vi "DualEncodersReadoutCore(NI-DAQmx).vi"(8 "error in":errorcluster, 9 "Position Out Queue":refnum<queue>, 10 "ctrl queue in":refnum<queue>) -> (0 "error out":errorcluster)   [LabVIEW 2014, in "EncoderReadout(NI-DAQmx).lvlib"]
uses:
  EncoderReadout(NI-DAQmx).lvlib
  VI/Encoder_State.ctl
  VI/EncoderReadout_Configs.ctl
  VI/EncoderReadout_PrivateStats.ctl
  <vilib>/Utility/error.llb/DialogType.ctl
  <vilib>/DAQmx/configure/timing.llb/DAQmx Timing (Sample Clock).vi
  <vilib>/DAQmx/read.llb/DAQmx Read (Counter 1D DBL 1Chan NSamp).vi
  <vilib>/Utility/error.llb/Error Cluster From Error Code.vi
  <vilib>/ErrorRing/Error Ring.xnode
  <resource>/objmgr/daqmx.rc
  <userlib>/Utility/ErrorLog_lib.lvlib
panel:
  out "ChangeDetect.Overflowed":bool
  out "start cts":i32
  out "TotalSampPerChanAcquired":dbl format="%#.2f"
  out "CurrReadPos":dbl
  out "AvailSampPerChan":u32
  out "PreGetPosition":dbl format="%_19f"
  out "flushbufffer":dbl format="%_19f"
  out "flush buffer":dbl[](graph)
  out "data":dbl[](graph)
  out "post flush buffer":i32
  out "pre-flush buffer":u32
  in  "SetPositionButton":bool
  out "elements":T1[](array[typedef])
  in  "Continuous":bool
  out "acqu. time":dbl
  out "pos get position":dbl format="%_19f"
  out "trans. start stamp":dbl format="%_19f"
  out "ctr_getpos":i32
  in  "SetPosition":dbl[](array[numeric])=[0.0, 0.0]
  in  "Get Configs":bool
  in  "StartAll":bool
  out "Core#":i32
  out "LiveStat":T2
  in  "EncoderReadout_Config":T3={"Mode"=enum."NSamples", "# Channels"=1, "# Samples"=128, "SyncSource"="/cDAQ1Mod3/PFI3", "Timeout (s)"=3600.0}
  out "Graph":dbl[][](graph)
  in  "Reset":bool
  in  "Close":bool
  in  "Open":bool
  in  "Quit":bool
  in  "GetPositions":bool
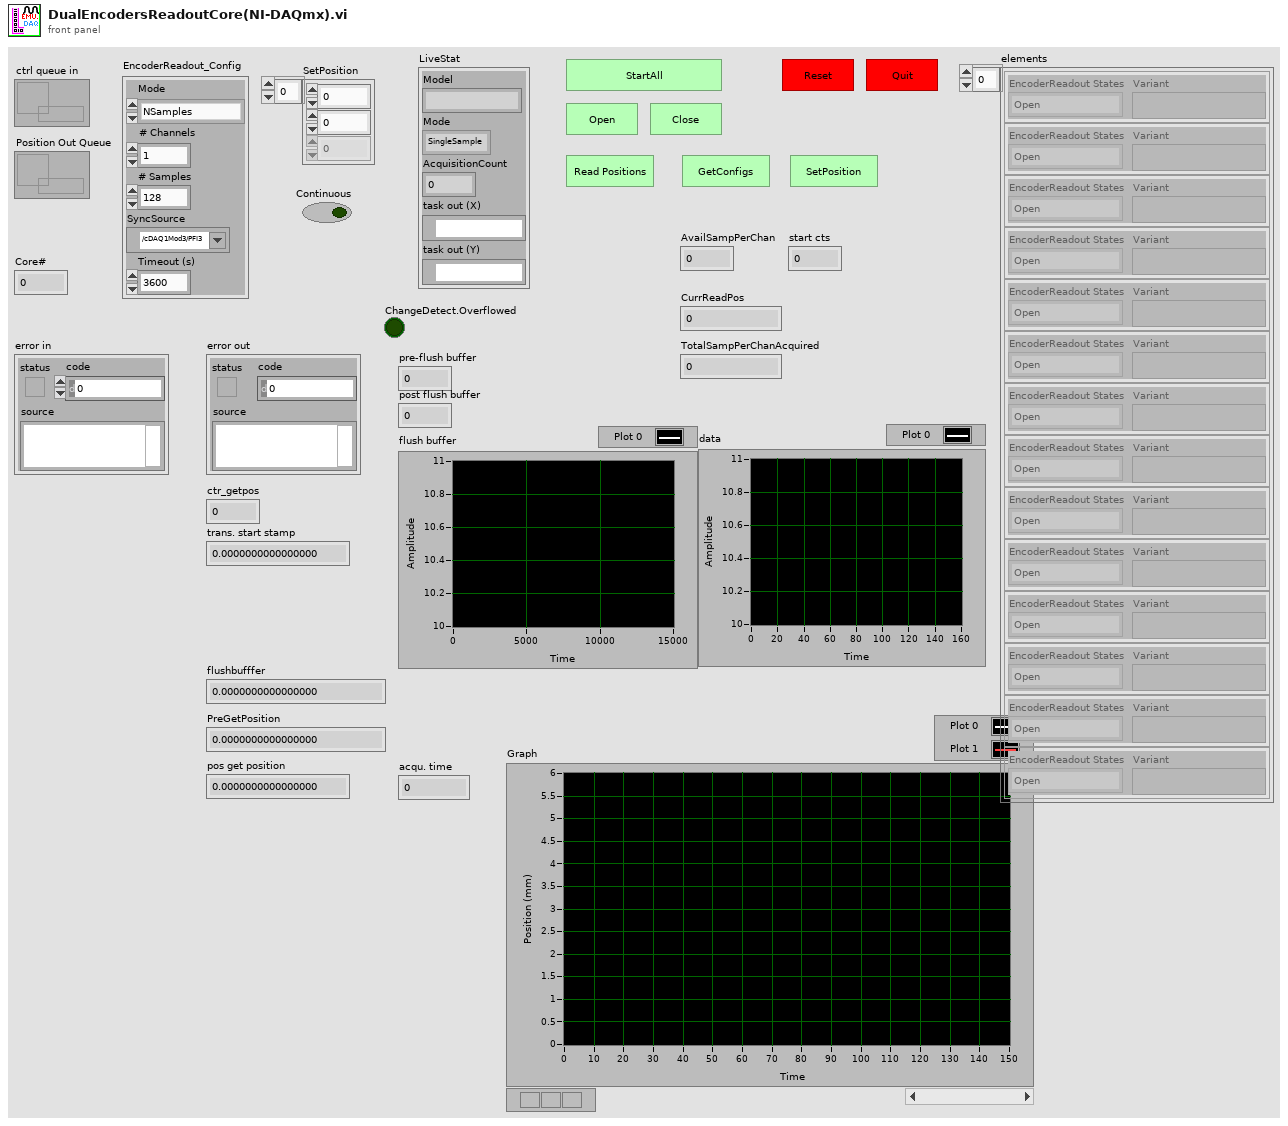
[diagram p1: front panel]
types:
  T1 = typedef "EncoderReadout(NI-DAQmx).lvlib/Encoder_State.ctl" = cluster{"EncoderReadout States":enum16{"Open", "Close", "Quit", "SetPosition", "SetPointsNum", "SetSyncChannel", "Start(Flush)", "GetPositions", "QueryStatus", "SetTimeout", "SetMode", "SetSignalOutputBuffer", "GetConfigs", "Wait", "Clear", "Stop", "FlushBuffer"}, "Variant":variant}
  T2 = typedef "EncoderReadout(NI-DAQmx).lvlib/EncoderReadout_PrivateStats.ctl" = cluster{"Model":string, "Mode":enum16{"SingleSample", "NSamples", "Continuous"}, "AcquisitionCount":i32, "task out (X)":refnum<k21>, "task out (Y)":refnum<k21>}
  T3 = typedef "EncoderReadout(NI-DAQmx).lvlib/EncoderReadout_Configs.ctl" = cluster{"Mode":enum16{"SingleSample", "NSamples", "Continuous"}, "# Channels":i32, "# Samples":i32, "SyncSource":tag, "Timeout (s)":dbl}
  T4 = typedef "DialogType.ctl" = u16
  T5 = cluster{"tickcount":u32, "Position":dbl[][], "Flag":enum16{"Normal", "MultiRecStart", "MultiRecEnd", "Reserved1", "Reserved2", "Reserved3"}}
  T6 = enum16{"Open", "Close", "Quit", "SetPosition", "SetPointsNum", "SetSyncChannel", "Start(Flush)", "GetPositions", "QueryStatus", "SetTimeout", "SetMode", "SetSignalOutputBuffer", "GetConfigs", "Wait", "Clear", "Stop", "FlushBuffer"}
  T7 = typedef "EncoderReadout_Configs.ctl" = cluster{"Mode":enum16{"SingleSample", "NSamples", "Continuous"}, "# Channels":i32, "# Samples":i32, "SyncSource":tag, "Timeout (s)":dbl}
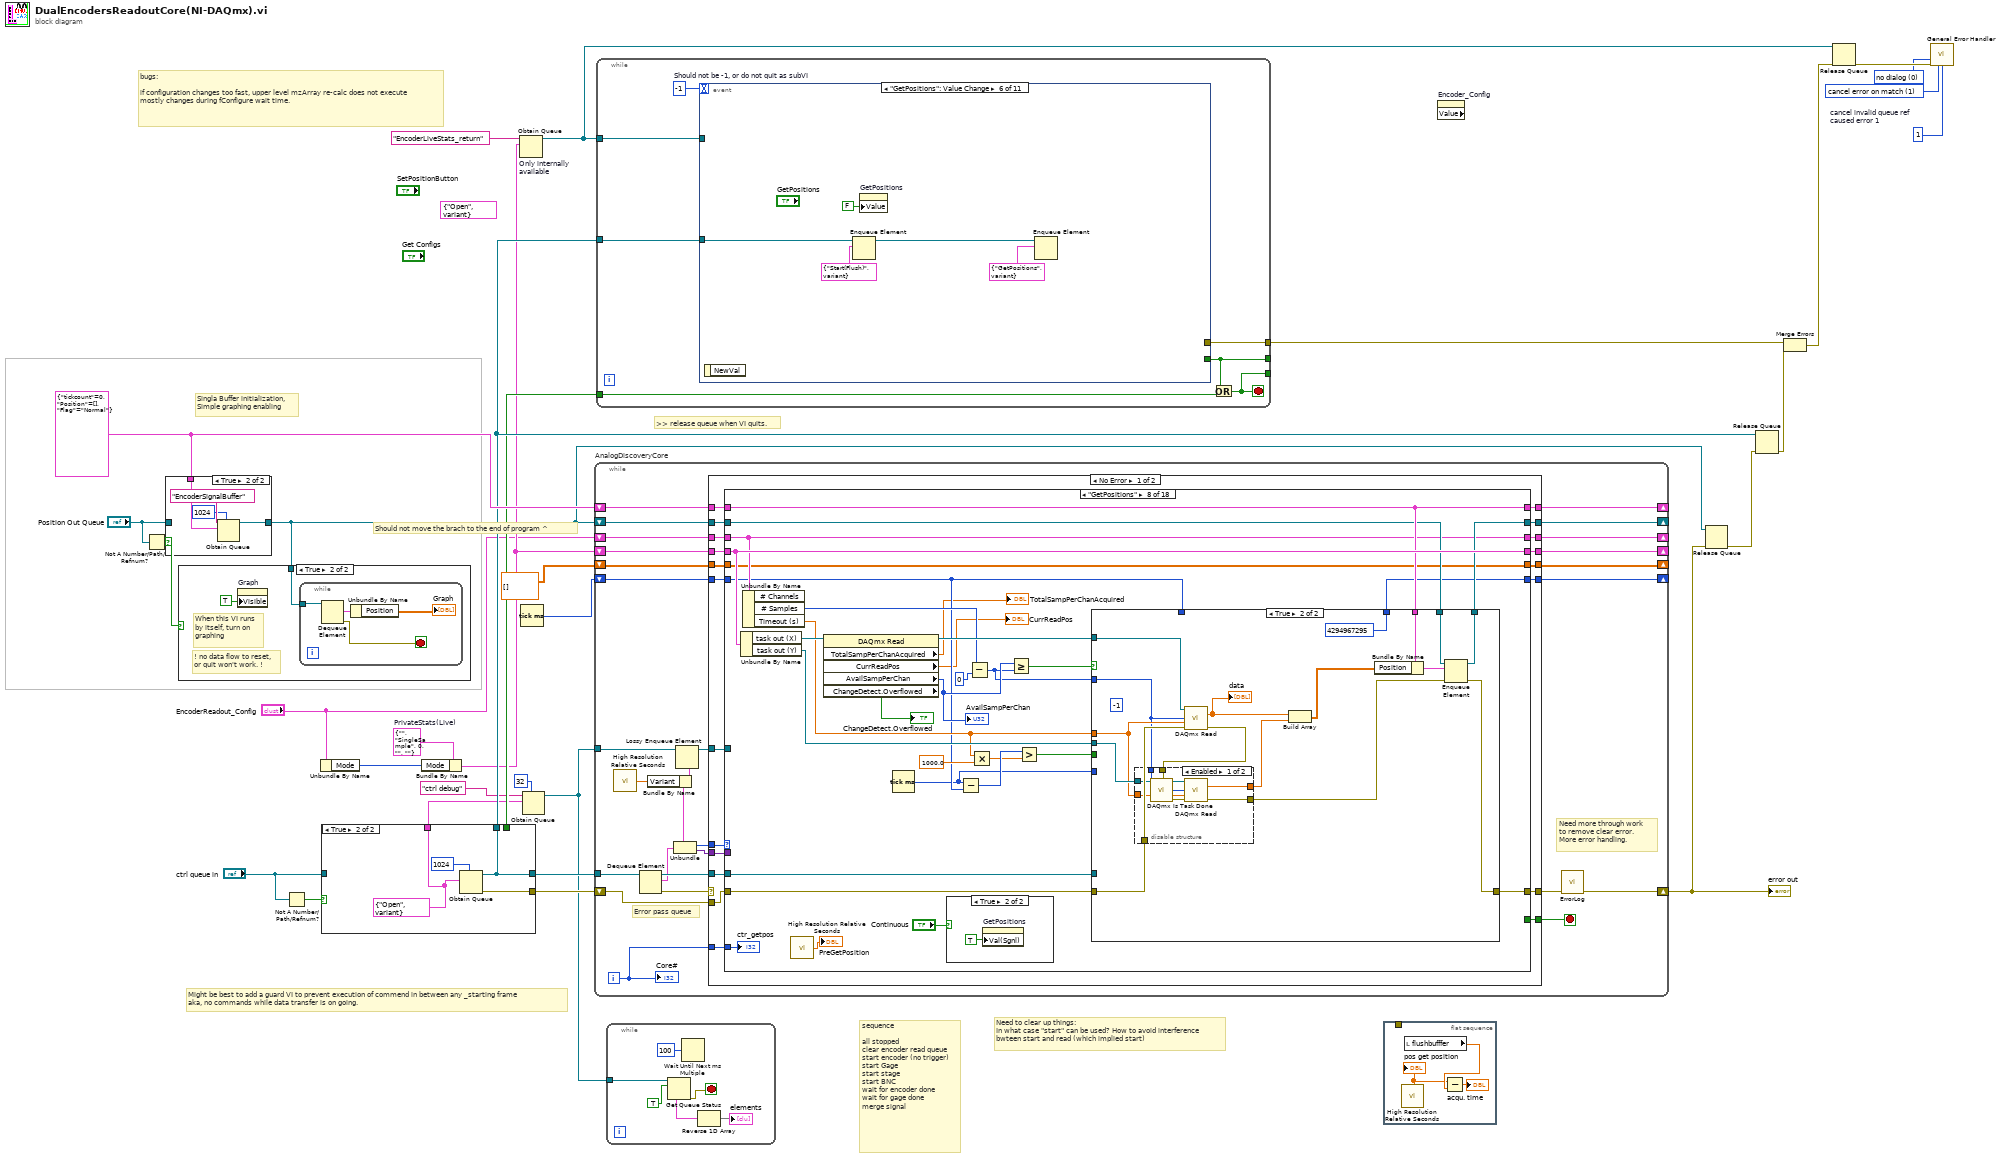
[diagram p0: block diagram]
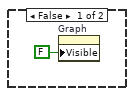
[diagram p2: hidden frame]
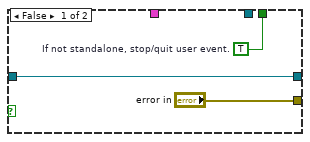
[diagram p4: hidden frame]
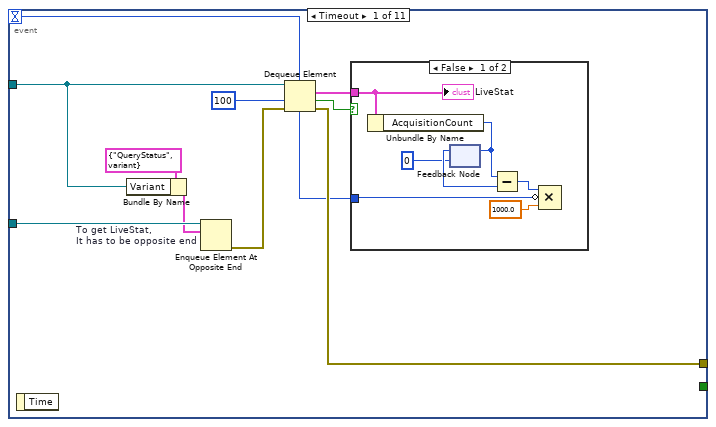
[diagram p5: hidden frame]
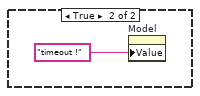
[diagram p6: hidden frame]
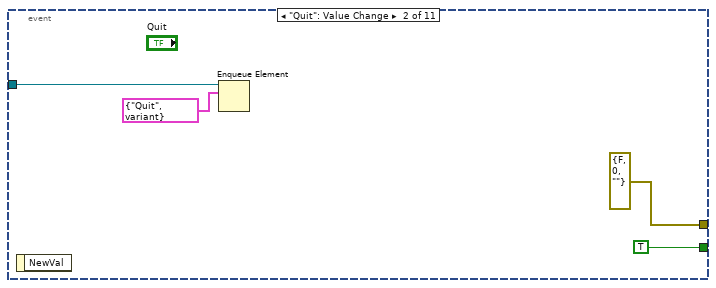
[diagram p7: hidden frame]
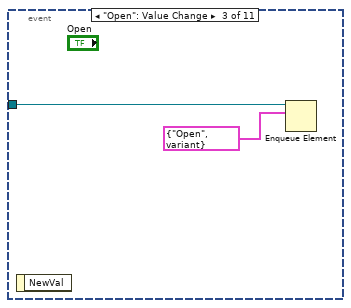
[diagram p8: hidden frame]
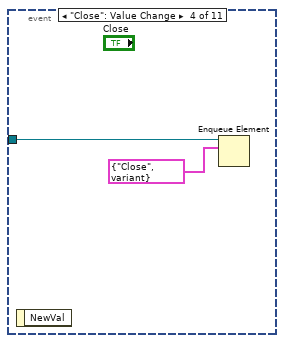
[diagram p9: hidden frame]
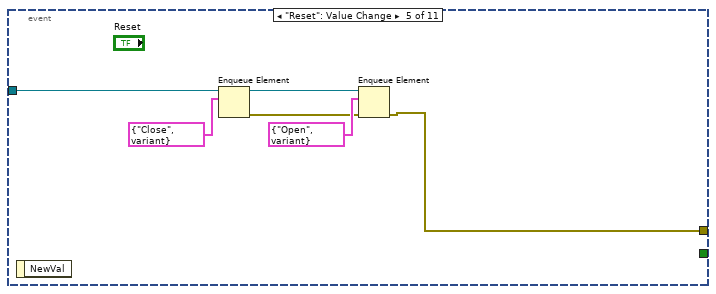
[diagram p10: hidden frame]
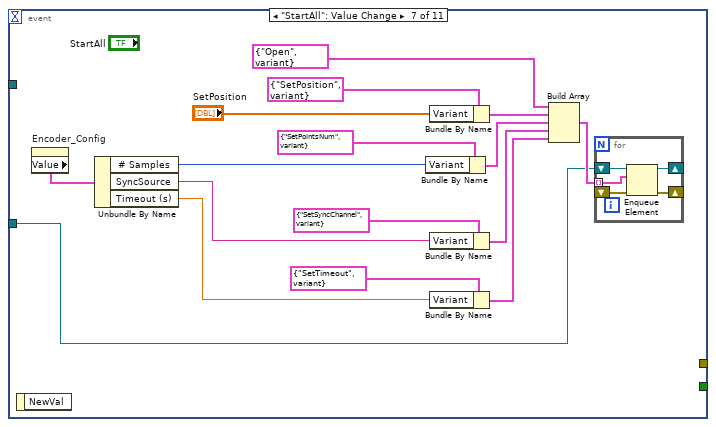
[diagram p11: hidden frame]
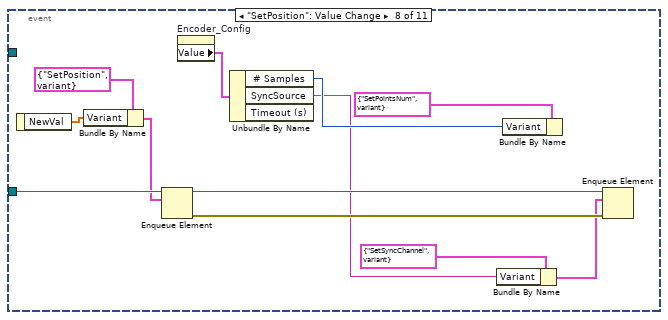
[diagram p12: hidden frame]
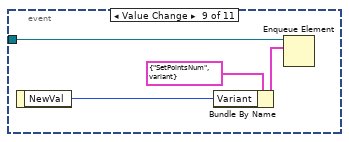
[diagram p13: hidden frame]
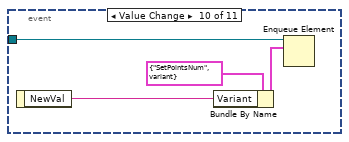
[diagram p14: hidden frame]
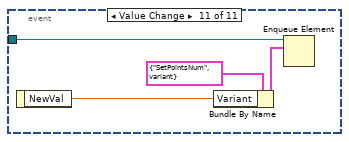
[diagram p15: hidden frame]
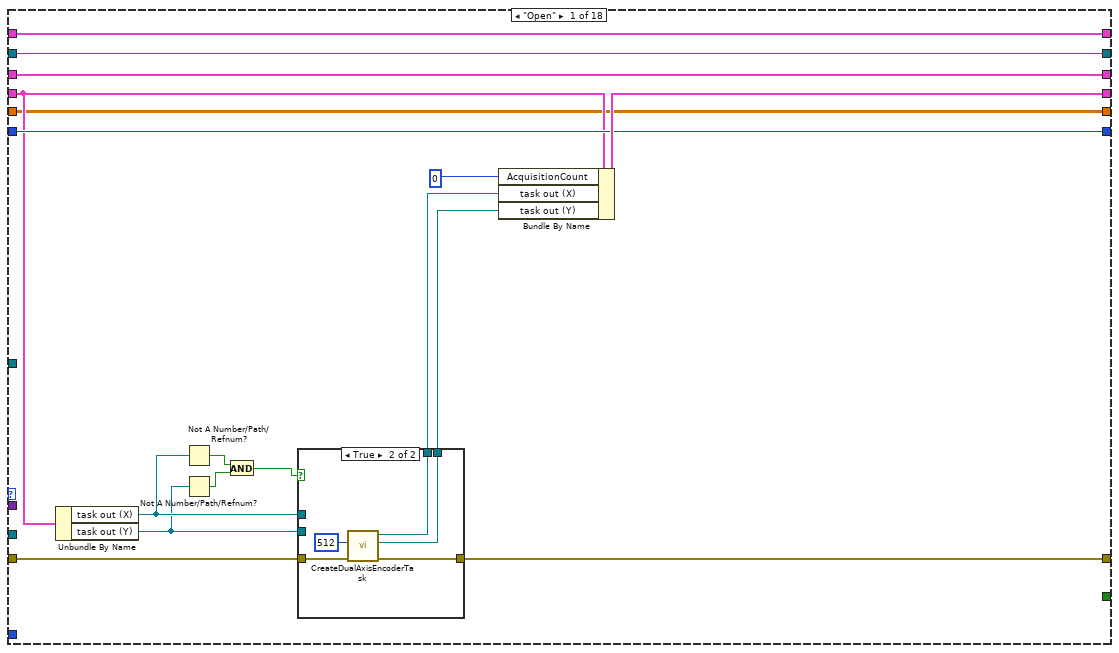
[diagram p16: hidden frame]
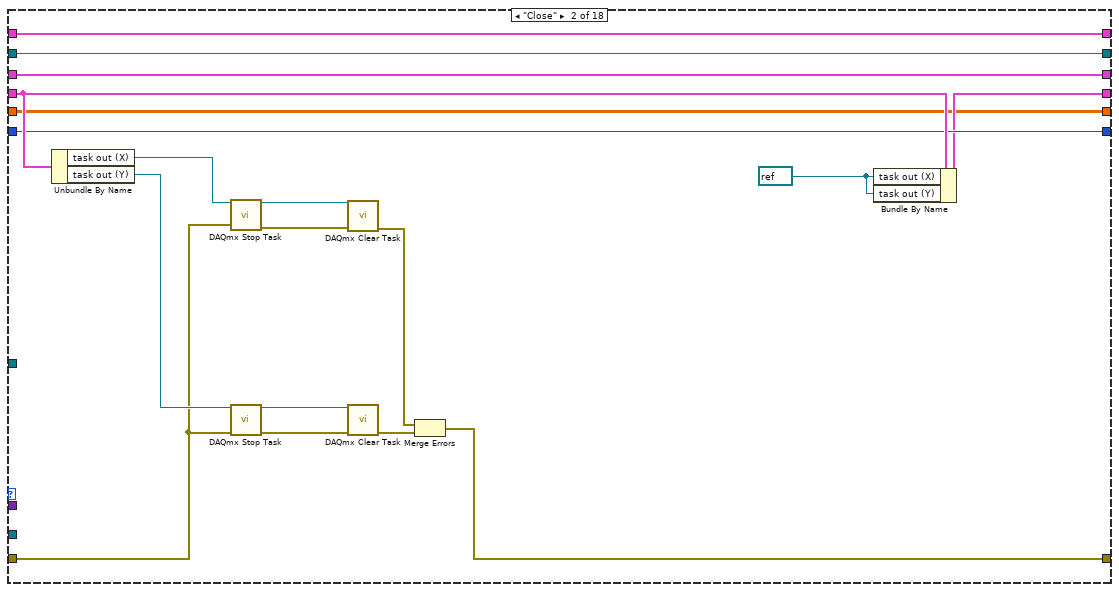
[diagram p18: hidden frame]
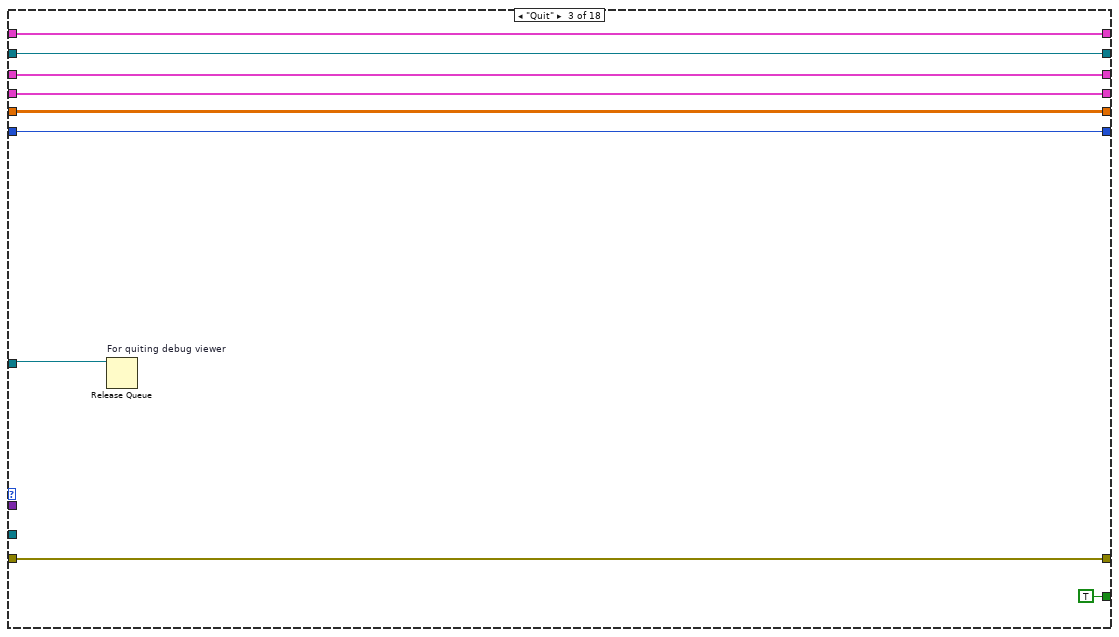
[diagram p19: hidden frame]
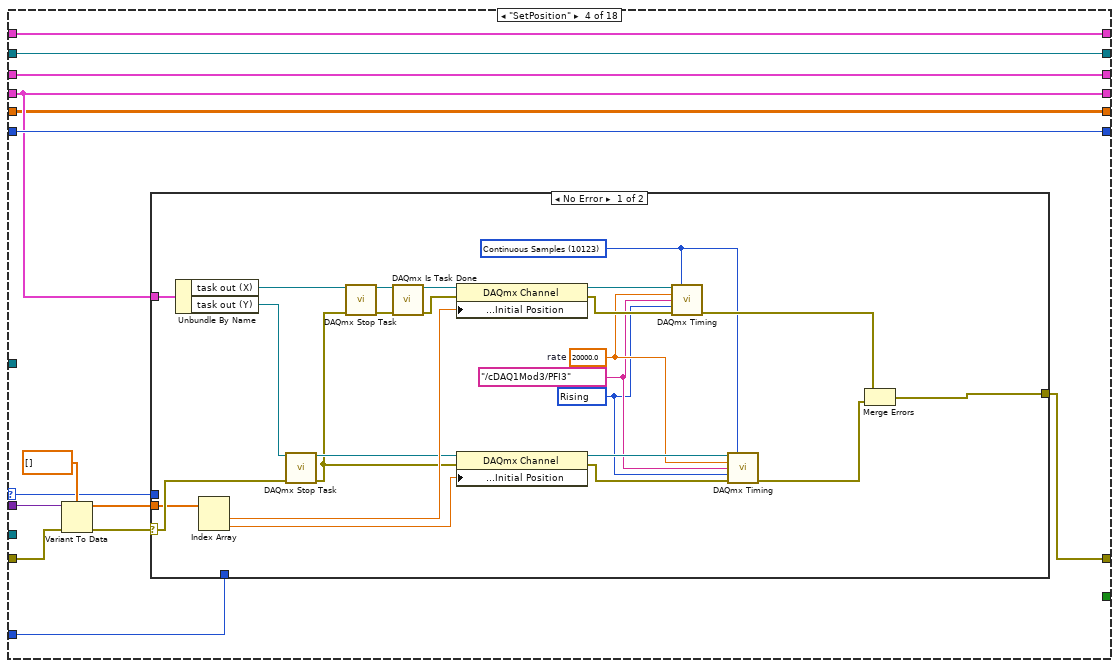
[diagram p20: hidden frame]
diagram:
  (unwired) T1 {"EncoderReadout States"=enum."Open", "Variant"=variant}
  w5 = T2 {"Model"="", "Mode"=enum."SingleSample", "AcquisitionCount"=0, "task out (X)"="", "task out (Y)"=""}  # PrivateStats(Live)
  w14 = 1  # cancel invalid queue ref caused error 1
  w15 = 1 items=["no exception", "cancel error on match", "set error on match"] ("[exception action] (none:0)")
  w16 = T4 0 items=["no dialog", "OK message", "continue or stop message", "OK message + warnings", "continue/stop + warnings"] ("type of dialog (OK msg:1)")
  w31 = T5 {"tickcount"=0, "Position"=[], "Flag"=enum."Normal"} ("Signal_Typedef")
  # "Need to clear up things:\nIn what case \"start\" can be used? How to avoid interference\nbwteen start and read (which implied start)"
  # "sequence\n\nall stopped\nclear encoder read queue\nstart encoder (no trigger)\nstart Gage\nstart stage\nstart BNC \nwait for encoder done\nwait for gage done\nmerge signal"
  # "Should not move the brach to the end of program ^"
  # "Might be best to add a guard VI to prevent execution of commend in between any _starting frame \naka, no commands while data transfer is on going."
  # "bugs:\n\nif configuration changes too fast, upper level mzArray re-calc does not execute\nmostly changes during fConfigure wait time."
  # "Singla Buffer initialization,\nSimple graphing enabling"
  # ">> release queue when VI quits."
  n1 = Not A Number/Path/Refnum?(number/path/refnum="Position Out Queue") -> (NaN/Path/Refnum?=w19:bool)
  n2 = case shown="True" w19 {
    tunnel: w31 -> [_ w36]
    tunnel: [w32 w33] -> w20
    tunnel: "Position Out Queue" -> [w32 _]
    frame False {
    }
    frame True {
      n3 = Obtain Queue(max queue size (-1, unlimited)=1024, name (unnamed)="EncoderSignalBuffer", element data type=w36) -> (queue out=w33:refnum<queue>)  [unwired: 2 in, 2 out]
    }
  }
  n4 = case shown="True" w19 {
    tunnel: w20 -> [_ w39]
    frame False {
      n5 = property on="Graph" class="WFGraph (strict)"("Visible"=FALSE) -> ()  [unwired: 2 in, 2 out]
    }
    frame True {
      # "! no data flow to reset,\nor quit won't work. !"
      # "When this VI runs\nby itself, turn on \ngraphing"
      n6 = property on="Graph" class="WFGraph (strict)"("Visible"=TRUE) -> ()  [unwired: 2 in, 2 out]
      n7 = while {
        tunnel: w39 -> [w43]
        stop <- w40 stop-if-true
        n8 = Dequeue Element(queue=w43) -> (element=w42:T5, error out=w40:errorcluster)  [unwired: 2 in, 2 out]
        n9 = Unbundle By Name(w42) -> ("Position"=→"Graph":dbl[][])
      }
    }
  }
  n10 = Not A Number/Path/Refnum?(number/path/refnum="ctrl queue in") -> (NaN/Path/Refnum?=w28:bool)
  n11 = Unbundle By Name("EncoderReadout_Config") -> ("Mode"=w10:enum16{"SingleSample", "NSamples", "Continuous"})
  n12 = case shown="True" w28 {
    tunnel: [w46 w47] -> w30
    tunnel: ["error in" w50] -> w29
    tunnel: "ctrl queue in" -> [w46 _]
    tunnel: [_ w47] -> w25
    tunnel: [w44 _] -> w13
    tunnel: [_ w48] -> w8
    frame False {
      w44 = TRUE  # If not standalone, stop/quit user event.
    }
    frame True {
      w48 = T1 {"EncoderReadout States"=enum."Open", "Variant"=variant}
      n13 = Obtain Queue(max queue size (-1, unlimited)=1024, element data type=w48) -> (queue out=w47:refnum<queue>, error out=w50:errorcluster)  [unwired: 3 in, 1 out]
    }
  }
  n14 = Bundle By Name(cluster=w5, "Mode"=w10) -> (w9:T2)
  n15 = Obtain Queue "Only internally\navailable"(name (unnamed)="EncoderLiveStats_return", element data type=w9) -> (queue out=w23:refnum<queue>)  [unwired: 3 in, 2 out]
  n16 = Tick Count (ms)() -> (millisecond timer value=w6:u32)
  n17 = Obtain Queue(max queue size (-1, unlimited)=32, name (unnamed)="ctrl debug", element data type=w8) -> (queue out=w3:refnum<queue>)  [unwired: 2 in, 2 out]
  n18 = while "AnalogDiscoveryCore" {
    shift-right: [w76] -> _
    shift-left: w20 -> [w77]
    tunnel: w30 -> [w65]
    shift-right: [w57] -> w18
    shift-left: w29 -> [w67]
    shift-right: [w74] -> _
    shift-left: "EncoderReadout_Config" -> [w73]
    shift-right: [w63] -> _
    shift-left: w9 -> [w72]
    shift-right: [w68] -> _
    shift-left: w31 -> [w71]
    shift-right: [w60] -> _
    shift-left: w6 -> [w61]
    shift-right: [w58] -> _
    shift-left: dbl[][] [] -> [w59]
    tunnel: w3 -> [w56]
    i -> [w52]
    stop <- w75 stop-if-true
    # "Need more through work\nto remove clear error.\nMore error handling."
    # "Error pass queue"
    n19 = call <vilib>:"High Resolution Relative Seconds.vi"() -> ("relative seconds"=w51:dbl)
    n20 = Dequeue Element(queue=w65) -> (queue out=w64:refnum<queue>, element=w55:T1, error out=w66:errorcluster)  [unwired: 2 in, 1 out]
    n21 = Bundle By Name(cluster=w55, "Variant"=w51) -> (w54:T1)
    n22 = Unbundle(w55) -> ("EncoderReadout States"=w70:T6, "Variant"=w69:variant)
    n23 = Lossy Enqueue Element(queue=w56, element=w54) -> (queue out=w53:refnum<queue>)  [unwired: 1 in, 3 out]
    n24 = case shown="No Error" w66 {
      tunnel: w77 -> [w97 w526]
      tunnel: [w96 w526] -> w76
      tunnel: [w95 TRUE] -> w75
      tunnel: [w94 w524] -> w62
      tunnel: [w93 w527] -> w74
      tunnel: w73 -> [w92 w527]
      tunnel: w72 -> [w91 w528]
      tunnel: w71 -> [w90 w525]
      tunnel: w64 -> [w89 _]
      tunnel: w70 -> [w88 _]
      tunnel: w69 -> [w87 _]
      tunnel: [w86 w525] -> w68
      tunnel: [w85 w528] -> w63
      tunnel: w67 -> [w84 _]
      tunnel: w61 -> [w83 w523]
      tunnel: [w82 w523] -> w60
      tunnel: w59 -> [w81 w522]
      tunnel: [w80 w522] -> w58
      tunnel: w52 -> [w79 _]
      tunnel: w53 -> [w78 _]
      frame No Error {
        n25 = case shown="\"GetPositions\"" w88 {
          selector: w88 -> [_ _ _ w153 w197 w228 _ _ _ _ _ _ _ _ _ _ _ w513]
          tunnel: w97 -> [w114 w140 w149 w163 w206 w237 w265 w313 w380 w393 w406 w414 w436 w450 w458 w470 w482 w521]
          tunnel: [w114 w140 w149 w163 w206 w237 w265 w312 w380 w393 w406 w415 w436 w450 w458 w470 w482 w521] -> w96
          tunnel: [_ _ TRUE _ _ _ _ _ _ _ _ _ _ _ _ _ _ _] -> w95
          tunnel: w89 -> [_ _ _ _ _ _ _ w308 _ _ _ _ _ _ _ _ _ _]
          tunnel: w84 -> [w106 w126 w145 w155 w199 w230 w264 w311 w375 w388 w397 w411 w428 w449 w457 w466 w480 w520]
          tunnel: [w107 w124 w145 w154 w198 w229 w263 w314 w374 w382 w398 w412 w429 w449 w457 w465 w478 w520] -> w94
          tunnel: [w105 w139 w148 w150 w193 w227 w261 w310 w373 w384 w405 w419 w430 w448 w456 w460 w486 w519] -> w93
          tunnel: w92 -> [w105 w139 w148 w150 w194 w227 w261 w310 w373 w383 w405 w419 w430 w448 w456 w460 w486 w519]
          tunnel: [w112 w131 w146 w157 w201 w232 w270 w316 w370 w391 w403 w418 w435 w447 w455 w467 w488 w518] -> w85
          tunnel: w91 -> [w104 w137 w146 w157 w201 w232 w270 w316 w370 w391 w402 w418 w435 w447 w455 w467 w488 w518]
          tunnel: w90 -> [w113 w138 w147 w162 w205 w236 w269 w315 w379 w392 w404 w417 w434 w446 w454 w469 w487 w517]
          tunnel: w87 -> [_ _ _ w160 w203 w234 _ _ w376 w390 w401 w416 w433 _ _ _ _ _]
          tunnel: [w113 w138 w147 w162 w205 w236 w269 w315 w379 w392 w404 w417 w434 w446 w454 w469 w487 w517] -> w86
          tunnel: w83 -> [w110 w136 w144 w161 w204 w235 w271 w294 w372 w387 w395 w408 w427 w445 w453 w468 w489 w516]
          tunnel: [w110 w136 w144 w161 w204 w235 w271 w297 w372 w387 w395 w408 w427 w445 w453 w468 w489 w516] -> w82
          tunnel: w81 -> [w98 w129 w142 w152 w195 w225 w266 w307 w369 w381 w394 w407 w425 w444 w452 w464 w483 w515]
          tunnel: [w98 w129 w142 w152 w195 w225 w266 w307 w369 w381 w394 w407 w425 w444 w452 w464 w483 w515] -> w80
          tunnel: w79 -> [_ _ _ w151 _ _ w262 w306 _ _ _ _ _ _ _ _ _ _]
          tunnel: w78 -> [_ _ w141 _ _ _ _ _ _ _ _ _ _ _ _ _ _ _]
          frame "Open" {
            n26 = Unbundle By Name(w104) -> ("task out (X)"=w100:refnum<k21>, "task out (Y)"=w99:refnum<k21>)
            n27 = Not A Number/Path/Refnum?(number/path/refnum=w100) -> (NaN/Path/Refnum?=w103:bool)
            n28 = Not A Number/Path/Refnum?(number/path/refnum=w99) -> (NaN/Path/Refnum?=w102:bool)
            n29 = And(x=w103, y=w102) -> (x .and. y?=w101:bool)
            n30 = case shown="True" w101 {
              tunnel: [w117 w122] -> w109
              tunnel: [w116 w121] -> w108
              tunnel: [w115 w120] -> w107
              tunnel: w106 -> [w115 w119]
              tunnel: w100 -> [w117 _]
              tunnel: w99 -> [w116 _]
              frame False {
              }
              frame True {
                n31 = call "CreateDualAxisEncoderTask.vi"("error in"=w119, "number of samples"=512) -> ("error out"=w120:errorcluster, "task out (Y)"=w121:refnum<k21>, "task out (X)"=w122:refnum<k21>)  [unwired: 7 in]
              }
            }
            n32 = Bundle By Name(cluster=w104, "AcquisitionCount"=0 ("TrigCount"), "task out (X)"=w109, "task out (Y)"=w108) -> (w112:T2)
          }
          frame "Close" {
            w130 = refnum<k21> refnum ("task out (X)")
            n33 = Unbundle By Name(w137) -> ("task out (X)"=w135:refnum<k21>, "task out (Y)"=w133:refnum<k21>)
            n34 = call <vilib>:"DAQmx Stop Task.vi"("task/channels in"=w135, "error in"=w126) -> ("task out"=w134:refnum<k21>, "error out"=w127:errorcluster)  [unwired: 12 in]
            n35 = call <vilib>:"DAQmx Stop Task.vi"("task/channels in"=w133, "error in"=w126) -> ("task out"=w128:refnum<k21>, "error out"=w125:errorcluster)  [unwired: 12 in]
            n36 = call <vilib>:"DAQmx Clear Task.vi"("task in"=w134, "error in"=w127) -> ("error out"=w123:errorcluster)  [unwired: 13 in]
            n37 = call <vilib>:"DAQmx Clear Task.vi"("task in"=w128, "error in"=w125) -> ("error out"=w132:errorcluster)  [unwired: 13 in]
            n38 = Merge Errors(w123, w132) -> (w124:errorcluster)
            n39 = Bundle By Name(cluster=w137, "task out (X)"=w130, "task out (Y)"=w130) -> (w131:T2)
          }
          frame "Quit" {
            n40 = Release Queue "For quiting debug viewer"(queue=w141) -> ()  [unwired: 2 in, 3 out]
          }
          frame "SetPosition" {
            n41 = Variant To Data(error in=w155, type=dbl[] [], Variant=w160) -> (data=w156:dbl[], error out=w158:errorcluster)
            n42 = case shown="No Error" w158 {
              selector: w158 -> [w181 w192]
              tunnel: w157 -> [w187 _]
              tunnel: w156 -> [w180 _]
              tunnel: [w171 w191] -> w154
              tunnel: w153 -> [_ w190]
              tunnel: w151 -> [_ _]
              frame No Error {
                w173 = 10123 items=["Finite Samples"=10178, "Continuous Samples"=10123, "Hardware Timed Single Point"=12522] ("sample mode")
                w175 = tag "/cDAQ1Mod3/PFI3" ("source")
                w176 = 20000.0  # rate
                w174 = 10280 items=["Rising"=10280, "Falling"=10171] ("active edge")
                n43 = Unbundle By Name(w187) -> ("task out (X)"=w183:refnum<k21>, "task out (Y)"=w182:refnum<k21>)
                n44 = Index Array(array=w180) -> (element #1=w179:dbl, element #2=w178:dbl)  [unwired: 2 in]
                n45 = call <vilib>:"DAQmx Stop Task.vi"("task/channels in"=w182, "error in"=w181) -> ("task out"=w165:refnum<k21>, "error out"=w164:errorcluster)  [unwired: 12 in]
                n46 = call <vilib>:"DAQmx Stop Task.vi"("task/channels in"=w183, "error in"=w164) -> ("task out"=w169:refnum<k21>, "error out"=w167:errorcluster)  [unwired: 12 in]
                n47 = call <vilib>:"DAQmx Is Task Done.vi"("task/channels in"=w169, "error in"=w167) -> ("task out"=w168:refnum<k21>, "error out"=w166:errorcluster)  [unwired: 11 in, 1 out]
                n48 = property class="DAQmx Channel"(reference=w168, error in=w166, "Counter Input:Position:Linear Encoder:Initial Position"=w179) -> (reference out=w185:refnum<k21>, error out=w184:errorcluster)
                n49 = property class="DAQmx Channel"(reference=w165, error in=w164, "Counter Input:Position:Linear Encoder:Initial Position"=w178) -> (reference out=w177:refnum<k21>, error out=w172:errorcluster)
                n50 = call-poly <vilib>:"DAQmx Timing.vi"("task/channels in"=w185, "sample mode"=w173, "rate"=w176, "source"=w175, "active edge"=w174, "error in"=w184) -> ("error out"=w186:errorcluster)  [unwired: 8 in, 1 out]
                n51 = call-poly <vilib>:"DAQmx Timing.vi"("task/channels in"=w177, "sample mode"=w173, "rate"=w176, "source"=w175, "active edge"=w174, "error in"=w172) -> ("error out"=w170:errorcluster)  [unwired: 8 in, 1 out]
                n52 = Merge Errors(w186, w170) -> (w171:errorcluster)
              }
              frame Error {
                n53 = Format Into String(initial string="Inernal error, inccorect \nvariant type.\nLocation: ", w190) -> (resulting string=w189:string)  [unwired: 2 in, 1 out]
                n54 = Bundle By Name(cluster=w192, "source"=w189) -> (w191:errorcluster)
              }
            }
          }
          frame "SetPointsNum" {
            n55 = Unbundle By Name(w194) -> ("# Samples"=w196:i32)
            n56 = Variant To Data(error in=w199, type=w196, Variant=w203) -> (data=w200:i32, error out=w202:errorcluster)
            n57 = case shown="No Error" w202 {
              selector: w202 -> [w215 w224]
              tunnel: w201 -> [w216 _]
              tunnel: w200 -> [w207 _]
              tunnel: [w215 w223] -> w198
              tunnel: w197 -> [_ w222]
              tunnel: w194 -> [w209 w219]
              tunnel: [w208 w219] -> w193
              frame No Error {
                n58 = Unbundle By Name(w216) -> ("task out (X)"=w214:refnum<k21>, "task out (Y)"=w213:refnum<k21>)
                n59 = In Range and Coerce(upper limit=1000000, x=w207, lower limit=2) -> (coerced(x)=w212:i32)  [unwired: 1 out]
                n60 = disable-structure shown="Enabled" {
                  disable-tunnel: w213 -> [w218 _]
                  disable-tunnel: w212 -> [w217 _]
                  frame Enabled {
                    n61 = property class="DAQmx Timing"(reference=w218, "SampQuant.SampPerChan"=w217) -> ()  [unwired: 1 in, 2 out]
                  }
                  frame Disabled {
                  }
                }
                n62 = property class="DAQmx Timing"(reference=w214, "SampQuant.SampPerChan"=w212) -> ()  [unwired: 1 in, 2 out]
                n63 = Bundle By Name(cluster=w209, "# Samples"=w207) -> (w208:T3)
                n64 = property on="# Samples" class="DigNum (strict)"("Value"=w207) -> ()  [unwired: 2 in, 2 out]
              }
              frame Error {
                n65 = Format Into String(initial string="Inernal error, inccorect \nvariant type.\nLocation: ", w222) -> (resulting string=w221:string)  [unwired: 2 in, 1 out]
                n66 = Bundle By Name(cluster=w224, "source"=w221) -> (w223:errorcluster)
              }
            }
          }
          frame "SetSyncChannel" {
            # "for references"
            n67 = Unbundle By Name(w227) -> ("SyncSource"=w226:tag)
            n68 = Variant To Data(error in=w230, type=w226, Variant=w234) -> (data=w231:tag, error out=w233:errorcluster)
            n69 = case shown="No Error" w233 {
              selector: w233 -> [w243 w255]
              tunnel: w232 -> [w244 _]
              tunnel: w231 -> [w240 _]
              tunnel: [w243 w254] -> w229
              tunnel: w228 -> [_ w253]
              frame No Error {
                n70 = Unbundle By Name(w244) -> ("task out (X)"=w242:refnum<k21>, "task out (Y)"=w241:refnum<k21>)
                n71 = disable-structure shown="Enabled" {
                  disable-tunnel: w241 -> [w250 _]
                  disable-tunnel: w240 -> [w249 _]
                  disable-tunnel: [w248 _] -> w238
                  frame Enabled {
                    n72 = property class="DAQmx Timing"(reference=w250, "SampClk.Src"=w249) -> (reference out=w248:refnum<k21>)  [unwired: 1 in, 1 out]
                  }
                  frame Disabled {
                  }
                }
                n73 = property class="DAQmx Timing"(reference=w242, "SampClk.Src"=w240) -> (reference out=w239:refnum<k21>)  [unwired: 1 in, 1 out]
                n74 = disable-structure shown="Enabled" {
                  disable-tunnel: w239 -> [w247 _]
                  disable-tunnel: w238 -> [w246 _]
                  frame Disabled {
                    w245 = 3 items=["verify"=2, "reserve"=4, "commit"=3, "unreserve"=5, "abort"=6] ("action")
                    n75 = call <vilib>:"DAQmx Control Task.vi"("task/channels in"=w247, "action"=w245) -> ()  [unwired: 12 in, 2 out]
                    n76 = call <vilib>:"DAQmx Control Task.vi"("task/channels in"=w246, "action"=w245) -> ()  [unwired: 12 in, 2 out]
                  }
                  frame Enabled {
                  }
                }
              }
              frame Error {
                n77 = Format Into String(initial string="Inernal error, inccorect \nvariant type.\nLocation: ", w253) -> (resulting string=w252:string)  [unwired: 2 in, 1 out]
                n78 = Bundle By Name(cluster=w255, "source"=w252) -> (w254:errorcluster)
              }
            }
          }
          frame "Start(Flush)" {
            # "Need to clear up things:\nIn what case \"start\" can be used? How to avoid interference\nbwteen start and read (which implied start)"
            n79 = Unbundle By Name(w261) -> ("# Channels"=w260:i32)
            n80 = Unbundle By Name(w270) -> ("task out (X)"=w268:refnum<k21>, "task out (Y)"=w267:refnum<k21>)
            n81 = case shown="2.." w260 {
              tunnel: [w276 w279] -> w258
              tunnel: w267 -> [w276 w278]
              tunnel: [_ w277] -> w257
              frame Default {
              }
              frame 2.. {
                n82 = disable-structure shown="Enabled" {
                  disable-tunnel: [w282 w284] -> w279
                  disable-tunnel: w278 -> [w281 w284]
                  disable-tunnel: [w280 _] -> w277
                  frame Enabled {
                    w283 = 4 items=["verify"=2, "reserve"=4, "commit"=3, "unreserve"=5, "abort"=6] ("action")
                    n83 = call <vilib>:"DAQmx Control Task.vi"("task/channels in"=w281, "action"=w283) -> ("task out"=w282:refnum<k21>, "error out"=w280:errorcluster)  [unwired: 12 in]
                  }
                  frame Disabled {
                  }
                }
              }
            }
            n84 = call <vilib>:"DAQmx Start Task.vi"("task/channels in"=w268, "error in"=w257) -> ("error out"=w259:errorcluster)  [unwired: 12 in, 1 out]
            n85 = case shown="2.." w260 {
              tunnel: w259 -> [w272 w275]
              tunnel: w258 -> [_ w274]
              tunnel: [w272 w273] -> w256
              frame Default {
              }
              frame 2.. {
                n86 = call <vilib>:"DAQmx Start Task.vi"("task/channels in"=w274, "error in"=w275) -> ("error out"=w273:errorcluster)  [unwired: 12 in, 1 out]
              }
            }
            n87 = Merge Errors(w256, w264) -> (w263:errorcluster)
            n88 = flat-sequence {
              tunnel: w263 -> [_]
              frame #0 {
                n89 = call <vilib>:"High Resolution Relative Seconds.vi"() -> ("relative seconds"=→"trans. start stamp":dbl)
              }
            }
            "start cts" <- w262
          }
          frame "GetPositions" {
            n90 = Unbundle By Name(w316) -> ("task out (X)"=w303:refnum<k21>, "task out (Y)"=w309:refnum<k21>)
            n91 = Unbundle By Name(w310) -> ("# Samples"=w299:i32, "Timeout (s)"=w296:dbl)  [unwired: 1 out]
            n92 = call <vilib>:"High Resolution Relative Seconds.vi"() -> ("relative seconds"=→"PreGetPosition":dbl)
            n93 = property class="DAQmx Read"(reference=w303) -> (reference out=w301:refnum<k21>, "TotalSampPerChanAcquired"=→"TotalSampPerChanAcquired":dbl, "CurrReadPos"=→"CurrReadPos":dbl, "AvailSampPerChan"=w300:u32, "ChangeDetect.Overflowed"=→"ChangeDetect.Overflowed":bool)  [unwired: 1 in, 1 out]
            "AvailSampPerChan" <- w300
            n94 = Tick Count (ms)() -> (millisecond timer value=w291:u32)
            n95 = case shown="True" "Continuous" {
              frame False {
              }
              frame True {
                n96 = property on="GetPositions" class="Bool (strict)"("Val(Sgnl)"=TRUE ("Value (Signaling)")) -> ()  [unwired: 2 in, 2 out]
              }
            }
            n97 = Subtract(x=w291, y=w294) -> (x-y=w293:u32)
            n98 = Subtract(x=w299, y=0) -> (x-y=w298:i32)
            n99 = Multiply(x=w296, y=1000.0) -> (x*y=w292:dbl)
            n100 = Greater Or Equal?(x=w300, y=w298) -> (x >= y?=w287:bool)
            n101 = Greater?(x=w293, y=w292) -> (0:w286:bool)
            n102 = case shown="True" w287 {
              tunnel: w315 -> [w322 w357]
              tunnel: [w330 w356] -> w314
              tunnel: w313 -> [w324 w355]
              tunnel: [w323 w354] -> w312
              tunnel: w311 -> [w330 w352]
              tunnel: w309 -> [w318 w351]
              tunnel: w308 -> [w332 _]
              tunnel: w296 -> [_ w349]
              tunnel: w298 -> [_ w346]
              tunnel: w301 -> [w321 w348]
              tunnel: w294 -> [w326 _]
              tunnel: [w328 u32 4294967295 ("millisecond timer value")] -> w297
              tunnel: w291 -> [w320 _]
              tunnel: w286 -> [_ _]
              frame False {
                # "not all data ready, continue waiting"
                n103 = Wait (ms)(milliseconds to wait=u32 250) -> ()  [unwired: 1 out]
                n104 = Equal?(x=u32 4294967295 ("millisecond timer value"), y=w326) -> (x = y?=w327:bool)
                n105 = case shown="True" FALSE {
                  tunnel: w324 -> [w333 w341]
                  tunnel: [w333 w340] -> w323
                  tunnel: w322 -> [_ w339]
                  tunnel: w321 -> [_ w338]
                  tunnel: w320 -> [_ _]
                  tunnel: w318 -> [_ w335]
                  frame False {
                  }
                  frame True {
                    # "THis frame is GARBAGE"
                    n106 = call-poly <vilib>:"DAQmx Read.vi"("task/channels in"=w338, "number of samples per channel"=-1) -> ("data"=w344:dbl[])  [unwired: 11 in, 2 out]
                    n107 = call-poly <vilib>:"DAQmx Read.vi"("task/channels in"=w335, "number of samples per channel"=-1) -> ("data"=w334:dbl[])  [unwired: 11 in, 2 out]
                    n108 = Build Array(w344, w334) -> (w342:dbl[][])
                    n109 = Bundle By Name(cluster=w339, "Position"=w342) -> (w343:T5)
                    n110 = Enqueue Element(queue=w341, element=w343) -> (queue out=w340:refnum<queue>)  [unwired: 2 in, 2 out]
                  }
                }
                n111 = Select(t=w320, s=w327, f=w326) -> (s? t:f=w328:u32)
                n112 = Enqueue Element At Opposite End(queue=w332, element=T1 {"EncoderReadout States"=enum."GetPositions", "Variant"=variant}) -> ()  [unwired: 2 in, 3 out]
              }
              frame True {
                (unwired) -1
                n113 = call-poly <vilib>:"DAQmx Read.vi"("task/channels in"=w348, "number of samples per channel"=w346, "timeout"=w349, "error in"=w352) -> ("data"=w360:dbl[], "error out"=w345:errorcluster)  [unwired: 9 in, 1 out]
                "data" <- w360
                n114 = disable-structure shown="Enabled" {
                  disable-tunnel: [w367 _] -> w359
                  disable-tunnel: [w366 w368] -> w353
                  disable-tunnel: w352 -> [_ w368]
                  disable-tunnel: w346 -> [w365 _]
                  disable-tunnel: w351 -> [w364 _]
                  disable-tunnel: w349 -> [w363 _]
                  disable-tunnel: w345 -> [w362 _]
                  frame Enabled {
                    n115 = call <vilib>:"DAQmx Is Task Done.vi"("task/channels in"=w364) -> ("task out"=w361:refnum<k21>)  [unwired: 12 in, 2 out]
                    n116 = call-poly <vilib>:"DAQmx Read.vi"("task/channels in"=w361, "number of samples per channel"=w365, "timeout"=w363, "error in"=w362) -> ("data"=w367:dbl[], "error out"=w366:errorcluster)  [unwired: 9 in, 1 out]
                  }
                  frame Disabled {
                  }
                }
                n117 = Build Array(w360, w359) -> (w350:dbl[][])
                n118 = Bundle By Name(cluster=w357, "Position"=w350) -> (w358:T5)
                n119 = Enqueue Element(queue=w355, element=w358, error in (no error)=w353) -> (queue out=w354:refnum<queue>, error out=w356:errorcluster)  [unwired: 1 in, 1 out]
              }
            }
            "ctr_getpos" <- w306
          }
          frame "QueryStatus" {
            n120 = Variant To Data(error in=w375, type=refnum<queue> refnum ("queue out"), Variant=w376) -> (data=w378:refnum<queue>, error out=w377:errorcluster)
            n121 = Enqueue Element "Send Core Stat"(queue=w378, element=w370, error in (no error)=w377) -> (error out=w374:errorcluster)  [unwired: 1 in, 2 out]
          }
          frame "SetTimeout" {
            n122 = Unbundle By Name(w383) -> ("Timeout (s)"=w389:dbl)
            n123 = Variant To Data(error in=w388, type=w389, Variant=w390) -> (data=w386:dbl, error out=w382:errorcluster)
            n124 = Bundle By Name(cluster=w383, "Timeout (s)"=w386) -> (w385:T3)
            n125 = Select(t=w383, s=w382, f=w385) -> (s? t:f=w384:T3)
          }
          frame "SetMode" {
            n126 = Unbundle By Name(w402) -> ("Mode"=w400:enum16{"SingleSample", "NSamples", "Continuous"})
            n127 = Variant To Data(error in=w397, type=w400, Variant=w401) -> (data=w399:enum16{"SingleSample", "NSamples", "Continuous"}, error out=w398:errorcluster)
            n128 = Select(t=w400, s=w398, f=w399) -> (s? t:f=w396:enum16{"SingleSample", "NSamples", "Continuous"})
            n129 = Bundle By Name(cluster=w402, "Mode"=w396) -> (w403:T2)
          }
          frame "SetSignalOutputBuffer" {
            n130 = Variant To Data(type=w414, Variant=w416) -> (data=w413:refnum<queue>, error out=w410:errorcluster)  [unwired: 1 in]
            n131 = Select(t=w414, s=w410, f=w413) -> (s? t:f=w415:refnum<queue>)
            n132 = xnode "Error Ring"() -> ("error out"=w409:errorcluster)
            n133 = Select(t=w409, s=w410, f=w411) -> (s? t:f=w412:errorcluster)
          }
          frame "GetConfigs" {
            n134 = Variant To Data(type=refnum<queue> refnum ("queue out"), Variant=w433) -> (data=w432:refnum<queue>, error out=w431:errorcluster)  [unwired: 1 in]
            n135 = case shown="No Error" w431 {
              selector: w431 -> [_ w442]
              tunnel: w432 -> [w440 _]
              tunnel: w430 -> [w437 _]
              tunnel: [w439 w442] -> w429
              tunnel: w428 -> [w438 _]
              frame No Error {
                n136 = Enqueue Element(queue=w440, element=w437, error in (no error)=w438) -> (error out=w439:errorcluster)  [unwired: 1 in, 2 out]
              }
              frame Error {
                n137 = One Button Dialog(message="Internal error in \"GetConfig_\"\nWrong type for querystatus.\nNo response sent, outer loop will wait forever.\nCheck caller syntax to fix it. ") -> ()  [unwired: 1 in, 1 out]
              }
            }
          }
          frame "Wait" {
            n138 = One Button Dialog(message="Not Implemented yet : \"Wait\" in Encoder readout") -> ()  [unwired: 1 in, 1 out]
          }
          frame "Clear" {
            # "Not implemented yet"
            n139 = One Button Dialog(message="Not Implemented yet : \"Clear\" in Encoder readout") -> ()  [unwired: 1 in, 1 out]
          }
          frame "Stop" {
            n140 = Unbundle By Name(w460) -> ("# Channels"=w459:i32)
            n141 = Unbundle By Name(w467) -> ("task out (X)"=w461:refnum<k21>, "task out (Y)"=w463:refnum<k21>)
            n142 = Build Array(w461, w463) -> (w462:refnum<k21>[])
            n143 = for {
              N: w459 -> [_]
              tunnel: w462 -> [w473] mode=indexing
              shift-right: [w472] -> w465
              shift-left: w466 -> [w471]
              n144 = call <vilib>:"DAQmx Stop Task.vi"("task/channels in"=w473, "error in"=w471) -> ("error out"=w472:errorcluster)  [unwired: 12 in, 1 out]
            }
          }
          frame "FlushBuffer" {
            # "to avoid error -201133"
            # "Need to clear up things:\nIn what case \"start\" can be used? How to avoid interference\nbwteen start and read (which implied start)"
            n145 = Unbundle By Name(w488) -> ("task out (X)"=w485:refnum<k21>, "task out (Y)"=w484:refnum<k21>)
            n146 = flat-sequence {
              tunnel: w485 -> [w493]
              tunnel: w484 -> [w499]
              tunnel: [w498] -> w476
              tunnel: [w497] -> w475
              tunnel: [w508] -> w474
              tunnel: [w509] -> w481
              tunnel: w476 -> [w509]
              tunnel: w475 -> [w508]
              frame #0 {
                w496 = 5.0
                # "Flush the position buffer on NI DAQ"
                n147 = property class="DAQmx Read"(reference=w493) -> (reference out=w491:refnum<k21>, error out=w490:errorcluster, "AvailSampPerChan"=w492:u32)  [unwired: 1 in]
                "pre-flush buffer" <- w492
                n148 = disable-structure shown="Enabled" {
                  disable-tunnel: w499 -> [w502 _]
                  disable-tunnel: [w505 _] -> w497
                  disable-tunnel: w496 -> [w504 _]
                  disable-tunnel: w490 -> [w500 _]
                  frame Enabled {
                    n149 = property class="DAQmx Read"(reference=w502, error in=w500) -> (reference out=w503:refnum<k21>, "AvailSampPerChan"=w501:u32)  [unwired: 1 out]
                    n150 = call-poly <vilib>:"DAQmx Read.vi"("task/channels in"=w503, "number of samples per channel"=w501, "timeout"=w504) -> ("error out"=w505:errorcluster)  [unwired: 10 in, 2 out]
                  }
                  frame Disabled {
                  }
                }
                n151 = call-poly <vilib>:"DAQmx Read.vi"("task/channels in"=w491, "number of samples per channel"=w492, "timeout"=w496) -> ("data"=w494:dbl[], "error out"=w498:errorcluster)  [unwired: 10 in, 1 out]
                "flush buffer" <- w494
                n152 = Array Size(array=w494) -> (size(s)=→"post flush buffer":i32)
              }
              frame #1 {
                n153 = call <vilib>:"High Resolution Relative Seconds.vi"() -> ("relative seconds"=→"flushbufffer":dbl)
                n154 = Wait (ms)(milliseconds to wait=u32 0) -> ()  [unwired: 1 out]
              }
            }
            n155 = Merge Errors(w481, w474, w480) -> (w479:errorcluster)
            n156 = call <vilib>:"Clear Errors.vi"("error in (no error)"=w479, "specific error code to clear (0: all)"=-200279) -> ("error out"=w478:errorcluster)  [unwired: 4 in, 1 out]
          }
          frame Default {
            n157 = Format Into String(w513) -> (resulting string=w511:string)  [unwired: 3 in, 1 out]
            n158 = Concatenate Strings("Not Implemented yet.  : " ("message"), w511, "in Encoder Readout" ("string")) -> (w512:string)
            n159 = One Button Dialog(message=w512) -> ()  [unwired: 1 in, 1 out]
          }
        }
      }
      frame Error {
        n160 = xnode "Error Ring"() -> ("error out"=w524:errorcluster)
      }
    }
    n161 = call <userlib>:"ErrorLog.vi"("error in (no error)"=w62) -> ("error out"=w57:errorcluster)  [unwired: 10 in]
    "Core#" <- w52
  }
  "error out" <- w18
  n162 = while {
    tunnel: w25 -> [w541]
    tunnel: w23 -> [w539]
    tunnel: w13 -> [w538]
    tunnel: [w537] -> w11
    tunnel: [w536] -> _
    tunnel: [w535] -> _
    stop <- w535 stop-if-true
    w540 = -1  # Should not be -1, or do not quit as subVI
    n163 = event shown="[5] \"GetPositions\": Value Change" {
      selector: _ -> [_ _ _ _ _ _ _ _ _ _ _]
      dyn-events: _ -> [_ _ _ _ _ _ _ _ _ _ _]
      timeout: w540 -> [w544 _ _ _ _ _ _ _ _ _ _]
      tunnel: w541 -> [w551 w563 w565 w567 w573 w578 w593 w609 w615 w619 w623]
      tunnel: w539 -> [w550 _ _ _ _ _ _ _ _ _ _]
      tunnel: [_ TRUE _ _ _ _ _ _ _ _ _] -> w536
      tunnel: [w549 errorcluster {"status"=FALSE, "code"=0, "source"=""} ("error constant") _ _ w568 _ _ _ _ _ _] -> w537
      event Timeout {
        n164 = event-data() -> ()  [unwired: 1 in, 1 out]
        n165 = Bundle By Name(cluster=T1 {"EncoderReadout States"=enum."QueryStatus", "Variant"=variant}, "Variant"=w550) -> (w548:T1)
        n166 = Enqueue Element At Opposite End "To get LiveStat,\nIt has to be opposite end"(queue=w551, element=w548) -> (error out=w547:errorcluster)  [unwired: 2 in, 2 out]
        n167 = Dequeue Element(queue=w550, timeout in ms (-1)=100, error in (no error)=w547) -> (element=w546:T2, timed out?=w545:bool, error out=w549:errorcluster)  [unwired: 1 out]
        n168 = case shown="False" w545 {
          tunnel: w546 -> [w552 _]
          tunnel: w544 -> [w555 _]
          frame False {
            n169 = Unbundle By Name(w552) -> ("AcquisitionCount"=w558:i32)
            n170 = feedback-in #1(w558) -> ()
            n171 = feedback #1(0 ("TrigCount")) -> (w557:i32)
            n172 = Subtract(x=w558, y=w557) -> (x-y=w556:i32)
            n173 = Compound Arithmetic op=MULTIPLY(w556, invert w555, 1000.0 ("value")) -> ()  [unwired: 1 out]
            "LiveStat" <- w552
          }
          frame True {
            n174 = property on="Model" class="Str"("Value"="timeout !" ("Model")) -> ()  [unwired: 2 in, 2 out]
          }
        }
      }
      event "Quit": Value Change {
        n175 = event-data() -> ()  [unwired: 1 in, 1 out]
        n176 = Enqueue Element(queue=w563, element=T1 {"EncoderReadout States"=enum."Quit", "Variant"=variant}) -> ()  [unwired: 2 in, 3 out]
      }
      event "Open": Value Change {
        n177 = event-data() -> ()  [unwired: 1 in, 1 out]
        n178 = Enqueue Element(queue=w565, element=T1 {"EncoderReadout States"=enum."Open", "Variant"=variant}) -> ()  [unwired: 2 in, 3 out]
      }
      event "Close": Value Change {
        n179 = event-data() -> ()  [unwired: 1 in, 1 out]
        n180 = Enqueue Element(queue=w567, element=T1 {"EncoderReadout States"=enum."Close", "Variant"=variant}) -> ()  [unwired: 2 in, 3 out]
      }
      event "Reset": Value Change {
        n181 = event-data() -> ()  [unwired: 1 in, 1 out]
        n182 = Enqueue Element(queue=w573, element=T1 {"EncoderReadout States"=enum."Close", "Variant"=variant}) -> (queue out=w570:refnum<queue>, error out=w569:errorcluster)  [unwired: 2 in, 1 out]
        n183 = Enqueue Element(queue=w570, element=T1 {"EncoderReadout States"=enum."Open", "Variant"=variant}, error in (no error)=w569) -> (error out=w568:errorcluster)  [unwired: 1 in, 2 out]
      }
      event "GetPositions": Value Change {
        n184 = event-data() -> ()  [unwired: 1 in, 1 out]
        n185 = Enqueue Element(queue=w578, element=T1 {"EncoderReadout States"=enum."Start(Flush)", "Variant"=variant}) -> (queue out=w575:refnum<queue>)  [unwired: 2 in, 2 out]
        n186 = property on="GetPositions" class="Bool (strict)"("Value"=FALSE ("GetPositions")) -> ()  [unwired: 2 in, 2 out]
        n187 = Enqueue Element(queue=w575, element=T1 {"EncoderReadout States"=enum."GetPositions", "Variant"=variant}) -> ()  [unwired: 2 in, 3 out]
      }
      event "StartAll": Value Change {
        n188 = event-data() -> ()  [unwired: 1 in, 1 out]
        n189 = property on="Encoder_Config" class="Clust (strict)"() -> ("Value"=w582:T7)  [unwired: 2 in, 2 out]
        n190 = Unbundle By Name(w582) -> ("# Samples"=w581:i32, "SyncSource"=w580:tag, "Timeout (s)"=w579:dbl)
        n191 = Bundle By Name(cluster=T1 {"EncoderReadout States"=enum."SetPointsNum", "Variant"=variant}, "Variant"=w581) -> (w588:T1)
        n192 = Bundle By Name(cluster=T1 {"EncoderReadout States"=enum."SetPosition", "Variant"=variant}, "Variant"="SetPosition") -> (w590:T1)
        n193 = Bundle By Name(cluster=T1 {"EncoderReadout States"=enum."SetSyncChannel", "Variant"=variant}, "Variant"=w580) -> (w585:T1)
        n194 = Bundle By Name(cluster=T1 {"EncoderReadout States"=enum."SetTimeout", "Variant"=variant}, "Variant"=w579) -> (w584:T1)
        n195 = Build Array(T1 {"EncoderReadout States"=enum."Open", "Variant"=variant}, w590, w588, w585, w584) -> (w594:T1[])
        n196 = for {
          shift-right: [w598] -> _
          shift-left: w593 -> [w599]
          tunnel: w594 -> [w597] mode=indexing
          shift-right: [w596] -> _
          shift-left: _ -> [w595]
          n197 = Enqueue Element(queue=w599, element=w597, error in (no error)=w595) -> (queue out=w598:refnum<queue>, error out=w596:errorcluster)  [unwired: 1 in, 1 out]
        }
      }
      event "SetPosition": Value Change {
        n198 = event-data() -> ("NewVal"=w610:dbl[])  [unwired: 1 in]
        n199 = Bundle By Name(cluster=T1 {"EncoderReadout States"=enum."SetPosition", "Variant"=variant}, "Variant"=w610) -> (w608:T1)
        n200 = Enqueue Element(queue=w609, element=w608) -> (queue out=w605:refnum<queue>, error out=w606:errorcluster)  [unwired: 2 in, 1 out]
        n201 = property on="Encoder_Config" class="Clust (strict)"() -> ("Value"=w603:T7)  [unwired: 2 in, 2 out]
        n202 = Unbundle By Name(w603) -> ("# Samples"=w604:i32, "SyncSource"=w601:tag)  [unwired: 1 out]
        n203 = Bundle By Name(cluster=T1 {"EncoderReadout States"=enum."SetSyncChannel", "Variant"=variant}, "Variant"=w601) -> (w600:T1)
        n204 = Bundle By Name(cluster=T1 {"EncoderReadout States"=enum."SetPointsNum", "Variant"=variant}, "Variant"=w604) -> ()  [unwired: 1 out]
        n205 = Enqueue Element(queue=w605, element=w600, error in (no error)=w606) -> ()  [unwired: 1 in, 3 out]
      }
      event Value Change {
        n206 = event-data() -> ("NewVal"=w613:i32)  [unwired: 1 in]
        n207 = Bundle By Name(cluster=T1 {"EncoderReadout States"=enum."SetPointsNum", "Variant"=variant}, "Variant"=w613) -> (w614:T1)
        n208 = Enqueue Element(queue=w615, element=w614) -> ()  [unwired: 2 in, 3 out]
      }
      event Value Change {
        n209 = event-data() -> ("NewVal"=w617:tag)  [unwired: 1 in]
        n210 = Bundle By Name(cluster=T1 {"EncoderReadout States"=enum."SetPointsNum", "Variant"=variant}, "Variant"=w617) -> (w618:T1)
        n211 = Enqueue Element(queue=w619, element=w618) -> ()  [unwired: 2 in, 3 out]
      }
      event Value Change {
        n212 = event-data() -> ("NewVal"=w621:dbl)  [unwired: 1 in]
        n213 = Bundle By Name(cluster=T1 {"EncoderReadout States"=enum."SetPointsNum", "Variant"=variant}, "Variant"=w621) -> (w622:T1)
        n214 = Enqueue Element(queue=w623, element=w622) -> ()  [unwired: 2 in, 3 out]
      }
    }
    n215 = Or(x=w536, y=w538) -> (x .or. y?=w535:bool)
  }
  n216 = while {
    tunnel: w3 -> [w629]
    stop <- w625 stop-if-true
    n217 = Get Queue Status(queue=w629, return elements? (F)=TRUE) -> (error out=w625:errorcluster, elements=w628:T1[])  [unwired: 1 in, 6 out]
    n218 = Wait Until Next ms Multiple(millisecond multiple=u32 100) -> ()  [unwired: 1 out]
    n219 = Reverse 1D Array(array=w628) -> (reversed array=→"elements":T1[])
  }
  n220 = flat-sequence {
    tunnel: _ -> [_]
    frame #0 {
      n221 = call <vilib>:"High Resolution Relative Seconds.vi"() -> ("relative seconds"=w631:dbl)
      "pos get position" <- w631
      n222 = local read "flushbufffer"() -> (w632:dbl)
      n223 = Subtract(x=w631, y=w632) -> (x-y=→"acqu. time":dbl)
    }
  }
  n224 = property on="Encoder_Config" class="Clust (strict)" props=["Value"]() -> ()  [unwired: 2 in, 3 out]
  n225 = Release Queue(queue=w20, error in (no error)=w18) -> (error out=w24:errorcluster)  [unwired: 1 in, 2 out]
  n226 = Release Queue(queue=w25, error in (no error)=w24) -> (error out=w22:errorcluster)  [unwired: 1 in, 2 out]
  n227 = Merge Errors(w11, w22) -> (w12:errorcluster)
  n228 = Release Queue(queue=w23, error in (no error)=w12) -> (error out=w17:errorcluster)  [unwired: 1 in, 2 out]
  n229 = call <vilib>:"General Error Handler.vi"("type of dialog (OK msg:1)"=w16, "error in (no error)"=w17, "[exception action] (none:0)"=w15, "[exception code]"=w14) -> ()  [unwired: 7 in, 5 out]
